vi "IsWidthRingCompatible.vi"(8 "error in (no error)":errorcluster, 11 "Width":u32) -> (0 "error out":errorcluster)   [LabVIEW 2023]
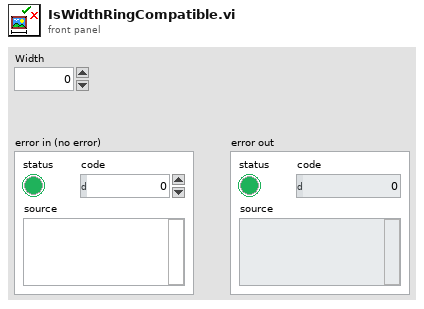
[diagram p1: front panel]
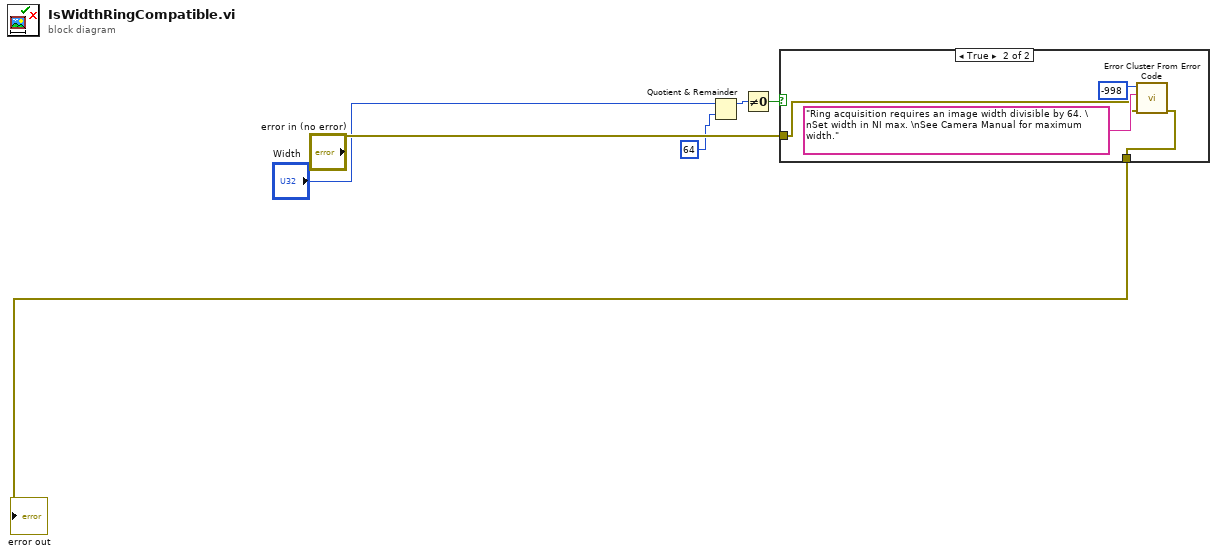
[diagram p0: block diagram]
diagram:
  n1 = Quotient & Remainder(x="Width", y=u32 64) -> (x-y*floor(x/y)=w4:u32)  [unwired: 1 out]
  n2 = Not Equal To 0?(x=w4) -> (x != 0?=w3:bool)
  n3 = case shown="True" w3 {
    tunnel: [w7 w8] -> w1
    tunnel: "error in (no error)" -> [w7 w9]
    frame False {
    }
    frame True {
      n4 = call <vilib>:"Error Cluster From Error Code.vi"("error in (no error)"=w9, "error message (\"\")"="Ring acquisition requires an image width divisible by 64. \nSet width in NI max. \nSee Camera Manual for maximum width." ("error message (\"\")"), "error code (0)"=-998) -> ("error out"=w8:errorcluster)  [unwired: 6 in]
    }
  }
  "error out" <- w1
